vi "Stop Core.vi"(10 "final error code":i32, 11 "ServiceManager-DebugView in":refnum<class "ServiceManager-DebugView.lvclass">) -> (3 "ServiceManager-DebugView out":refnum<class "ServiceManager-DebugView.lvclass">)   [LabVIEW 2020, in "ServiceManager-DebugView.lvlib" / "ServiceManager-DebugView.lvclass"]
doc: "(<B>Filename</B>: Actor Framework.lvlib:Actor.lvclass:Stop Core.vi)\n\nDefines what the actor does before it stops. Use the <B>final error code</B> input to determine whether the actor shut down in response to an error.\n\nBy default, this method passes the Stop message along to all auto-stop nested actors. A descendant class may override this method to define additional behavior, such as shutting down any processes the actor initiated in its override of the Actor Core method."
uses:
  ServiceManager-DebugView.lvclass
  <vilib>/ActorFramework/Actor/Actor.lvclass
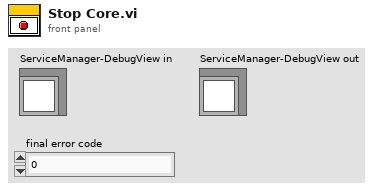
[diagram p1: front panel]
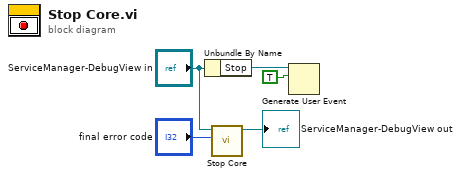
[diagram p0: block diagram]
diagram:
  n1 = Unbundle By Name("ServiceManager-DebugView in") -> ("Stop"=w2:refnum<user-event>)
  n2 = call-parent "Stop Core.vi"("final error code"="final error code", "Actor in"="ServiceManager-DebugView in") -> ("Actor out"=→"ServiceManager-DebugView out":refnum<class "ServiceManager-DebugView.lvclass">)  [unwired: 9 in]
  n3 = Generate User Event(user event=w2, event data cluster=TRUE ("event data")) -> ()  [unwired: 2 in, 2 out]
